vi "SizeUp.vi"() -> ()   [LabVIEW 2024, in "VarCircularBuffer.Tests.Units.lvlib"]
uses:
  VarCircularBuffer.Tests.Units.lvlib
  VarCircularBuffer.lvclass/VarCircularBuffer.ctl
  ReadCount.vi
  Sort.vi
  <vilib>/addons/_JKI Toolkits/Caraya/classes/Assert/Assert True.vi
  <vilib>/addons/_JKI Toolkits/Caraya/classes/Assert/Assert False.vi
  <vilib>/addons/_JKI Toolkits/Caraya/classes/Assert/Assert Equal Value and Type_Variant.vi
  <vilib>/addons/_JKI Toolkits/Caraya/classes/Assert/Assert Equal Value_Variant.vi
  <vilib>/addons/_JKI Toolkits/Caraya/classes/Assert/Assert.lvclass
  VarCircularBuffer.lvclass
  <vilib>/addons/_JKI Toolkits/Caraya/classes/Test/Test.lvclass
panel:
  in  "Size up Add Expected":variant[](array[variant])=[variant(i32 0), variant(i32 1), variant(i32 2), variant(i32 3), variant(i32 4), variant(i32 5), variant(i32 6), variant(i32 7), variant(i32 8), variant(i32 9), variant(i32 255)]
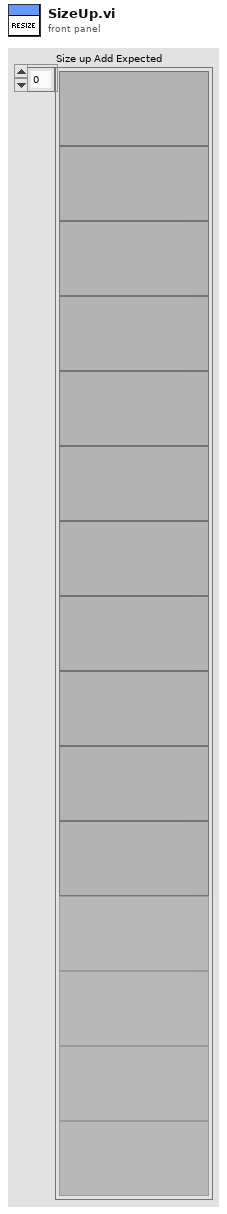
[diagram p1: front panel]
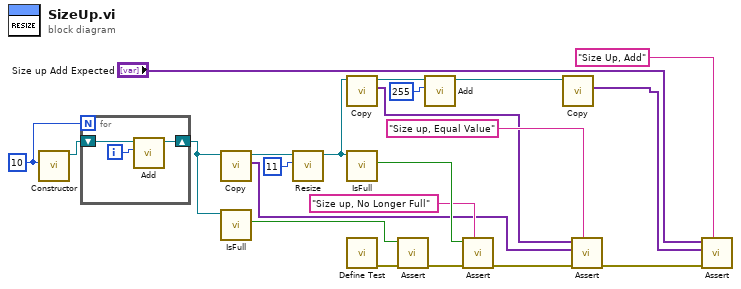
[diagram p0: block diagram]
diagram:
  w7 = u32 10 ("Capacity")
  n1 = call "Constructor.vi"("Capacity"=w7) -> ("TypedCircularBuffer out"=w6:refnum<class "VarCircularBuffer.lvclass">)  [unwired: 10 in]
  n2 = for {
    N: w7 -> [_]
    shift-right: [w24] -> w5
    shift-left: w6 -> [w25]
    i -> [w23]
    n3 = call "Add.vi"("Element"=w23, "TypedCircularBuffer in"=w25) -> ("TypedCircularBuffer out"=w24:refnum<class "VarCircularBuffer.lvclass">)  [unwired: 7 in, 2 out]
  }
  n4 = call "Copy.vi"("TypedCircularBuffer in"=w5) -> ("Copied Buffer"=w13:variant[], "TypedCircularBuffer out"=w18:refnum<class "VarCircularBuffer.lvclass">)  [unwired: 9 in]
  n5 = call "IsFull.vi"("TypedCircularBuffer in"=w5) -> ("Full?"=w21:bool)  [unwired: 9 in, 1 out]
  n6 = call "Resize.vi"("Capacity"=u32 11, "TypedCircularBuffer in"=w18) -> ("TypedCircularBuffer out"=w17:refnum<class "VarCircularBuffer.lvclass">)  [unwired: 9 in]
  n7 = call "Copy.vi"("TypedCircularBuffer in"=w17) -> ("Copied Buffer"=w1:variant[], "TypedCircularBuffer out"=w12:refnum<class "VarCircularBuffer.lvclass">)  [unwired: 9 in]
  n8 = call "IsFull.vi"("TypedCircularBuffer in"=w17) -> ("Full?"=w19:bool)  [unwired: 9 in, 1 out]
  n9 = call <vilib>:"Define Test.vi"() -> ("error out"=w4:errorcluster)  [unwired: 10 in, 1 out]
  n10 = call-poly <vilib>:"Assert.vi"("error in (no error)"=w4, "True?"=w21) -> ("error out"=w20:errorcluster)  [unwired: 8 in, 1 out]
  n11 = call "Add.vi"("Element"=u8 255, "TypedCircularBuffer in"=w12) -> ("TypedCircularBuffer out"=w10:refnum<class "VarCircularBuffer.lvclass">)  [unwired: 7 in, 2 out]
  n12 = call-poly <vilib>:"Assert.vi"("Label"="Size up, No Longer Full", "error in (no error)"=w20, "False?"=w19) -> ("error out"=w16:errorcluster)  [unwired: 7 in, 1 out]
  n13 = call "Copy.vi"("TypedCircularBuffer in"=w10) -> ("Copied Buffer"=w2:variant[])  [unwired: 9 in, 1 out]
  n14 = call-poly <vilib>:"Assert.vi"("Label"="Size up, Equal Value", "error in (no error)"=w16, "Y"=w13, "X"=w1) -> ("error out"=w3:errorcluster)  [unwired: 6 in, 1 out]
  n15 = call-poly <vilib>:"Assert.vi"("Label"="Size Up, Add", "error in (no error)"=w3, "Y"=w2, "X"="Size up Add Expected") -> ()  [unwired: 6 in, 2 out]
